vi "ddsSweepTimeArrayConvert.vi"(7 "Pre 3.0 AOM driver":bool, 9 "Register":dbl=7.0 min=0.0 max=15.0 step=1.0 format="%#.1f", 10 "Sweep Time Array (ms)":dbl[](array[numeric])=[1e-05] min=0.0 max=42000.0 step=1e-05 format="%.5f", 11 "Frequency Difference Array (MHz)":dbl[](array[numeric])=[0.0] min=0.0 max=180.0 step=8.3819e-08 format="%.7f") -> (1 "Characters for FPGA":string="L70100000001\r\n")   [LabVIEW 2013, in "DDS9954_v2013.lvlib"]
uses:
  DDS9954_v2013.lvlib
  dataToAscii_8bit.vi
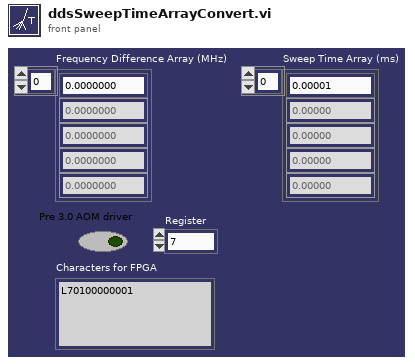
[diagram p1: front panel]
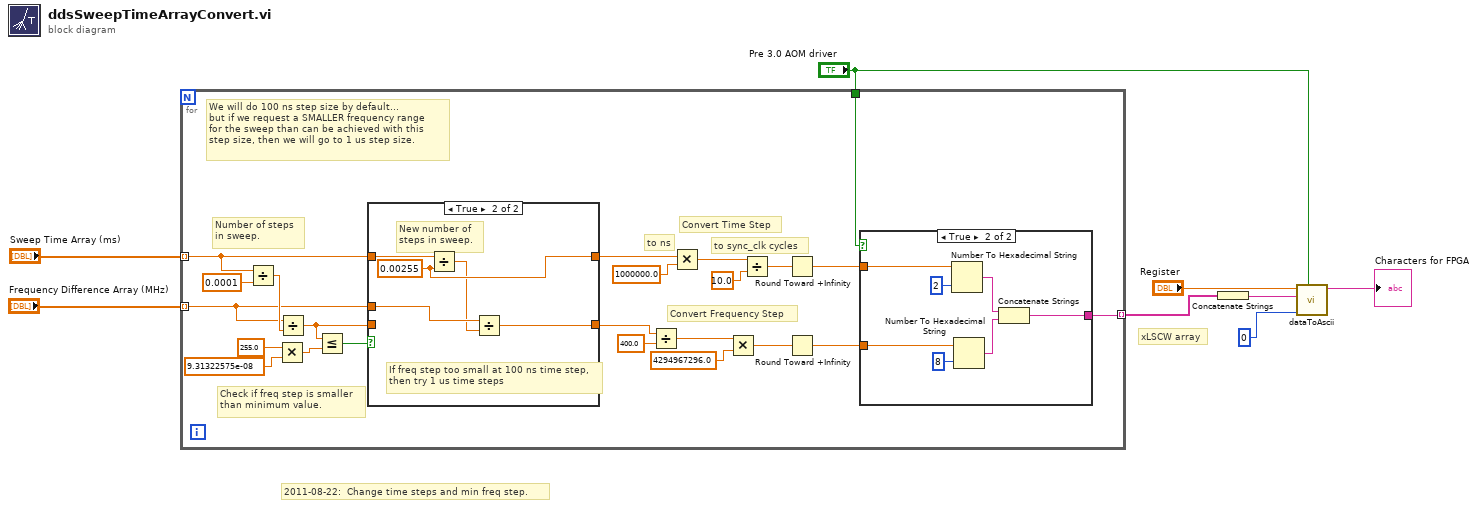
[diagram p0: block diagram]
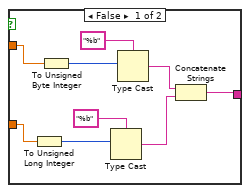
[diagram p2: hidden frame]
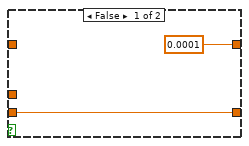
[diagram p3: hidden frame]
diagram:
  # "2011-08-22:  Change time steps and min freq step."
  # "xLSCW array"
  n1 = for {
    tunnel: "Sweep Time Array (ms)" -> [w28] mode=indexing
    tunnel: "Frequency Difference Array (MHz)" -> [w27] mode=indexing
    tunnel: [w13] -> w5 mode=indexing
    tunnel: "Pre 3.0 AOM driver" -> [w9]
    # "to sync_clk cycles"
    # "to ns"
    # "Convert Time Step"
    # "Convert Frequency Step"
    # "Check if freq step is smaller\nthan minimum value."
    # "Number of steps\nin sweep."
    # "We will do 100 ns step size by default...\nbut if we request a SMALLER frequency range\nfor the sweep than can be achieved with this\nstep size, then we will go to 1 us step size."
    n2 = Divide(x=w28, y=0.0001) -> (x/y=w29:dbl)
    n3 = Multiply(x=255.0 ("y"), y=9.31322575e-08) -> (x*y=w10:dbl)
    n4 = Divide(x=w27, y=w29) -> (x/y=w26:dbl)
    n5 = Less Or Equal?(x=w26, y=w10) -> (x <= y?=w30:bool)
    n6 = case shown="True" w30 {
      tunnel: w28 -> [_ w54]
      tunnel: w27 -> [_ w52]
      tunnel: [0.0001 ("y") w53] -> w15
      tunnel: w26 -> [w49 _]
      tunnel: [w49 w50] -> w14
      frame False {
      }
      frame True {
        w53 = 0.00255 ("y")
        # "New number of\nsteps in sweep."
        # "If freq step too small at 100 ns time step,\nthen try 1 us time steps"
        n7 = Divide(x=w54, y=w53) -> (x/y=w51:dbl)
        n8 = Divide(x=w52, y=w51) -> (x/y=w50:dbl)
      }
    }
    n9 = Divide(x=w14, y=400.0) -> (x/y=w18:dbl)
    n10 = Multiply(x=w15, y=1000000.0) -> (x*y=w21:dbl)
    n11 = Multiply(x=w18, y=4294967296.0) -> (x*y=w24:dbl)
    n12 = Divide(x=w21, y=10.0) -> (x/y=w22:dbl)
    n13 = Round Toward +Infinity(x=w22) -> (ceil(x): smallest int >= x=w23:dbl)
    n14 = Round Toward +Infinity(x=w24) -> (ceil(x): smallest int >= x=w25:dbl)
    n15 = case shown="True" w9 {
      tunnel: w25 -> [w33 w47]
      tunnel: w23 -> [w34 w46]
      tunnel: [w32 w45] -> w13
      frame False {
        n16 = To Unsigned Long Integer(number=w33) -> (unsigned 32bit integer=w37:u32)
        n17 = To Unsigned Byte Integer(number=w34) -> (unsigned 8bit integer=w39:u8)
        n18 = Type Cast(type="%b", x=w37) -> (*(type *) &x=w36:string)
        n19 = Type Cast(type="%b", x=w39) -> (*(type *) &x=w40:string)
        n20 = Concatenate Strings(w40, w36) -> (w32:string)
      }
      frame True {
        n21 = Number To Hexadecimal String(1:i16 2 ("width (-)"), 2:w46) -> (0:w43:string)
        n22 = Number To Hexadecimal String(1:i16 8 ("width (-)"), 2:w47) -> (0:w44:string)
        n23 = Concatenate Strings(w43, w44) -> (w45:string)
      }
    }
  }
  n24 = Concatenate Strings(w5) -> (w4:string)
  n25 = call-poly "dataToAscii.vi"("Pre 3.0 AOM driver version?"="Pre 3.0 AOM driver", "HEX min width (pre 3.0)"=u8 0, "Input String"=w4, "Register"="Register") -> ("Characters to FPGA"=→"Characters for FPGA":string)  [unwired: 7 in]
